vi "VISA wait.vi"(8 "error in (no error)":errorcluster, 11 "Cobolt in":refnum<class "Cobolt.lvclass">) -> (0 "error out":errorcluster, 3 "Cobolt out":refnum<class "Cobolt.lvclass">)   [LabVIEW 2012, in "Cobolt.lvclass"]
uses:
  Cobolt.lvclass
  Cobolt.lvclass/Cobolt.ctl
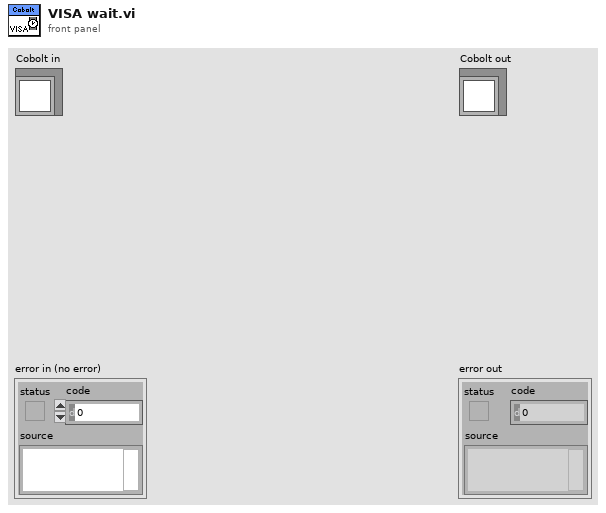
[diagram p1: front panel]
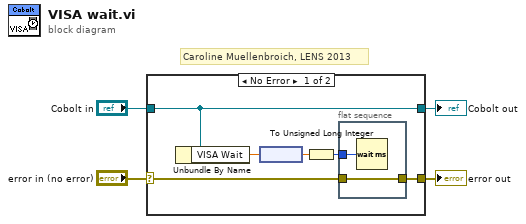
[diagram p0: block diagram]
diagram:
  # "Caroline Muellenbroich, LENS 2013"
  n1 = case shown="No Error" "error in (no error)" {
    selector: "error in (no error)" -> [w6 w14]
    tunnel: [w5 w14] -> w3
    tunnel: [w7 w13] -> w1
    tunnel: "Cobolt in" -> [w7 w13]
    frame No Error {
      n2 = Unbundle By Name(w7) -> ("VISA Wait"=w10:dbl[unit])
      n3 = node(w10) -> (w9:dbl)
      n4 = To Unsigned Long Integer(number=w9) -> (unsigned 32bit integer=w8:u32)
      n5 = flat-sequence {
        tunnel: w6 -> [w12]
        tunnel: [w12] -> w5
        tunnel: w8 -> [w11]
        frame #0 {
          n6 = Wait (ms)(milliseconds to wait=w11) -> ()  [unwired: 1 out]
        }
      }
    }
    frame Error {
    }
  }
  "error out" <- w3
  "Cobolt out" <- w1
